vi "Set Scale Name.vi"(8 "error in (no error)":errorcluster, 9 "name":string, 10 "index":i32, 11 "Scaling configuration in":refnum<class "Scaling configuration.lvclass">) -> (0 "error out":errorcluster, 3 "Scaling configuration out":refnum<class "Scaling configuration.lvclass">)   [LabVIEW 2015, in "Scaling configuration.lvclass"]
uses:
  Scaling configuration.lvclass
  Scaling configuration.lvclass/Scaling configuration.ctl
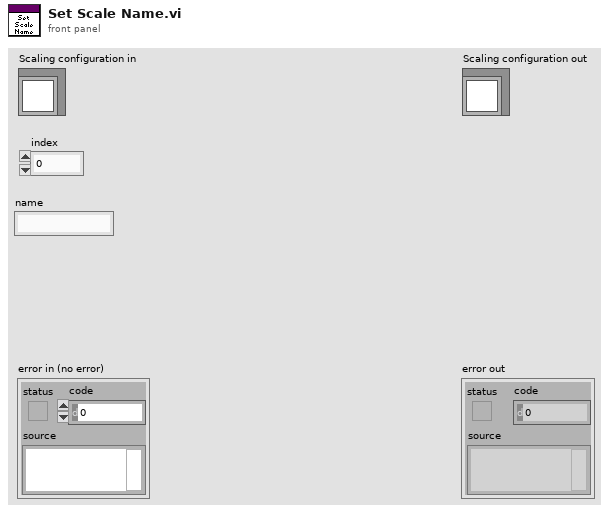
[diagram p1: front panel]
types:
  T1 = typedef "Scaling configuration.lvclass/scale data types.ctl" = enum16{"Double", "Single", "I64", "I32", "I16", "I8", "U64", "U32", "U16", "U8"}
  T2 = cluster{"mappings":cluster{"input channel":refnum<class "TBM channel.lvclass">, "output channel":refnum<class "TBM channel.lvclass">, "input data type":T1, "output data type":T1}[], "name":string}[]
  T3 = cluster{"mappings":cluster{"input channel":refnum<class "TBM channel.lvclass">, "output channel":refnum<class "TBM channel.lvclass">, "input data type":T1, "output data type":T1}[], "name":string}
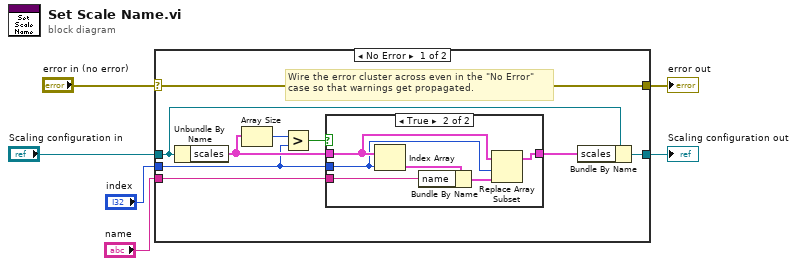
[diagram p0: block diagram]
diagram:
  n1 = case shown="No Error" "error in (no error)" {
    selector: "error in (no error)" -> [w15 w24]
    tunnel: [w15 w24] -> w5
    tunnel: [w9 w23] -> w3
    tunnel: "Scaling configuration in" -> [w10 w23]
    tunnel: "name" -> [w8 _]
    tunnel: "index" -> [w7 _]
    frame No Error {
      # "Wire the error cluster across even in the \"No Error\"\ncase so that warnings get propagated."
      n2 = Unbundle By Name(w10) -> ("scales"=w12:T2)
      n3 = Array Size(array=w12) -> (size(s)=w14:i32)
      n4 = Greater?(x=w14, y=w7) -> (0:w13:bool)
      n5 = case shown="True" w13 {
        tunnel: w12 -> [w16 w21]
        tunnel: w7 -> [_ w20]
        tunnel: w8 -> [_ w22]
        tunnel: [w16 w18] -> w11
        frame False {
        }
        frame True {
          n6 = Index Array(array=w21, index=w20) -> (element=w19:T3)
          n7 = Bundle By Name(cluster=w19, "name"=w22) -> (w17:T3)
          n8 = Replace Array Subset(array=w21, new element=w17, index=w20) -> (w18:T2)
        }
      }
      n9 = Bundle By Name(cluster=w10, "scales"=w11) -> (w9:refnum<class "Scaling configuration.lvclass">)
    }
    frame Error {
    }
  }
  "error out" <- w5
  "Scaling configuration out" <- w3
